vi "LabVIEW Load Cell Function.vi"() -> ()   [LabVIEW 2019]
uses:
  <vilib>/Analysis/baseanly.llb/Mean (DBL).vi
  <vilib>/Analysis/NI_AALBase.lvlib
panel:
  out "Right Cell":dbl format="%#_8f"
  out "Left Cell":dbl format="%#_8f"
  out "Combined Load":dbl format="%#_8f"
  in  "Filename":path=path "test.lvm"
  in  "Log data?":bool=TRUE caption="Enable"
  in  "OK Button":bool
  in  "Offest 2":dbl
  in  "Offset 1":dbl
  out "Waveform Chart":dynamicdata(graph)
  in  "stop (F)":bool
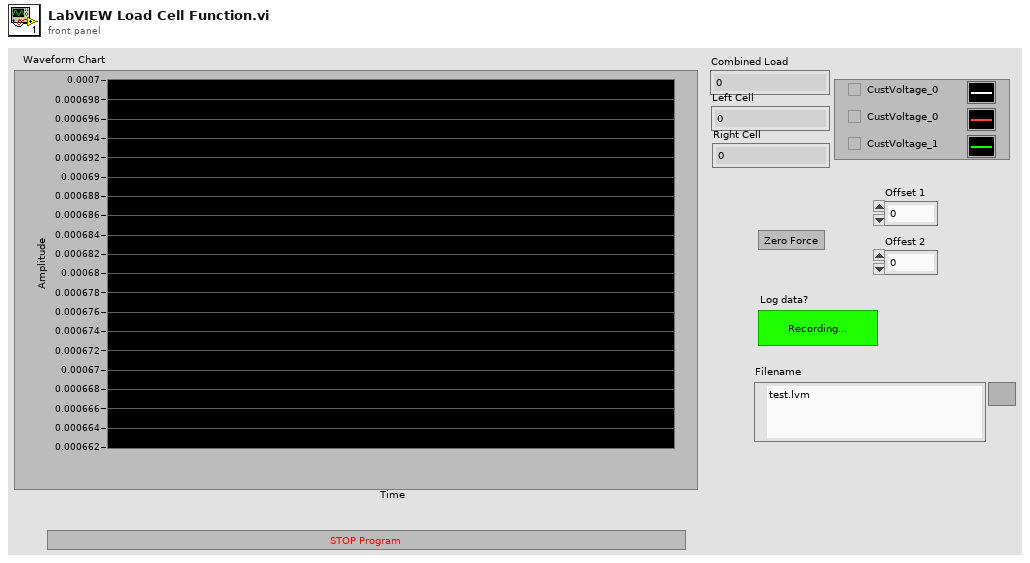
[diagram p1: front panel]
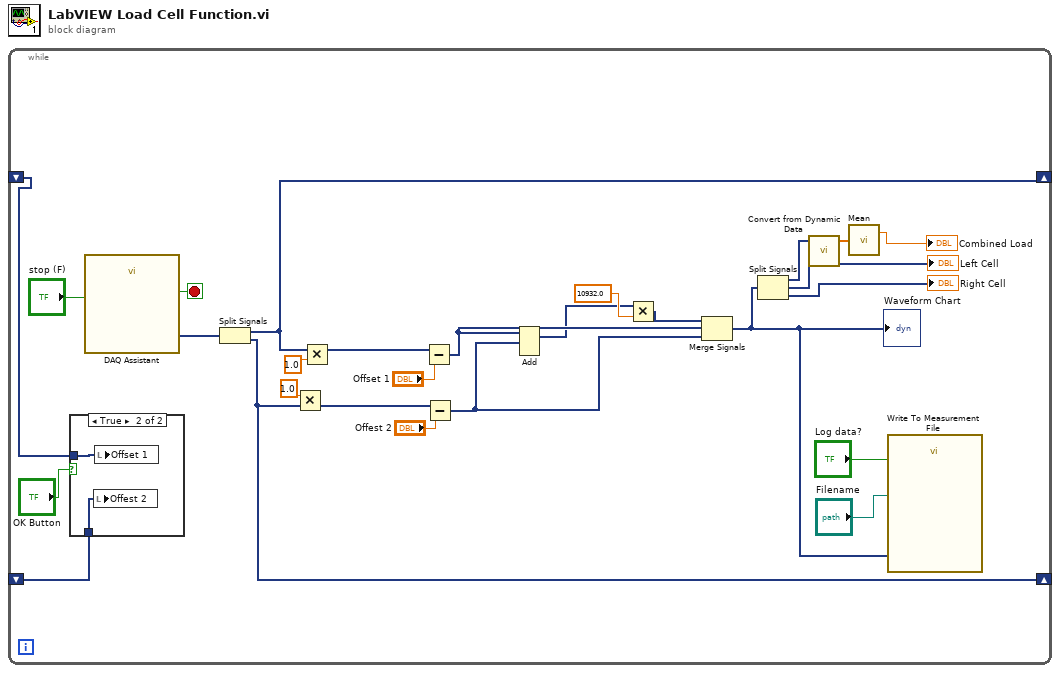
[diagram p0: block diagram]
diagram:
  n1 = while {
    shift-right: [w19] -> _
    shift-left: _ -> [w18]
    shift-right: [w20] -> _
    shift-left: _ -> [w17]
    stop <- w26 stop-if-true
    n2 = case shown="True" "OK Button" {
      tunnel: w18 -> [_ w29]
      tunnel: w17 -> [_ w28]
      frame False {
      }
      frame True {
        n3 = local write "Offest 2"(w29) -> ()
        n4 = local write "Offset 1"(w28) -> ()
      }
    }
    n5 = call "DAQ Assistant"("stop (F)"="stop (F)") -> ("data"=w25:dynamicdata, "stopped"=w26:bool)  [unwired: 15 in, 2 out]
    n6 = Split Signals(w25) -> (w20:dynamicdata, w19:dynamicdata)  [unwired: 2 in]
    n7 = Multiply(x=1.0, y=w19) -> (x*y=w12:dynamicdata)
    n8 = Multiply(x=w20, y=1.0) -> (x*y=w13:dynamicdata)
    n9 = Subtract(x=w13, y="Offset 1") -> (x-y=w21:dynamicdata)
    n10 = Subtract(x=w12, y="Offest 2") -> (x-y=w22:dynamicdata)
    n11 = Add(1:w22, 2:w21) -> (0:w8:dynamicdata)  [unwired: 1 in, 1 out]
    n12 = Multiply(x=w8, y=10932.0) -> (x*y=w7:dynamicdata)
    n13 = Merge Signals(w7, w21, w22) -> (w6:dynamicdata)
    "Waveform Chart" <- w6
    n14 = Split Signals(w6) -> (w4:dynamicdata, →"Left Cell":dynamicdata, →"Right Cell":dynamicdata)  [unwired: 3 in]
    n15 = call "Convert from Dynamic Data"("Dynamic Data Type"=w4) -> ("Array"=w3:dbl[])  [unwired: 3 in]
    n16 = call-poly <vilib>:"Mean.vi"("X"=w3) -> ("mean"=→"Combined Load":dbl)  [unwired: 1 out]
    n17 = call "Write To Measurement File"("Signals"=w6, "Enable"="Log data?", "Filename"="Filename") -> ()  [unwired: 14 in, 3 out]
  }
